vi "CAN Main.vi"(8 "error in (no error)":errorcluster, 10 "Interface":refnum<k21>="CAN1", 11 "Sequence Context In":refnum<k7>) -> (0 "error out":errorcluster)   [LabVIEW 2021, in "CAN wrapper.lvlib"]
uses:
  CAN wrapper.lvlib
  Private Controls/CAN States.ctl
  Private Controls/Setting.ctl
  <vilib>/addons/TestStand/_TSUtility.llb/TestStand - Set Property Value (Numeric Array).vi
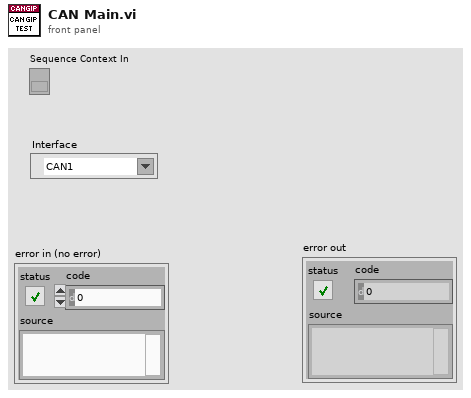
[diagram p1: front panel]
types:
  T1 = typedef "CAN wrapper.lvlib/CAN States.ctl" = enum16{"Init", "Rx Sess", "Tx Sess", "Read Signals", "Write Signals", "Close"}
  T2 = typedef "CAN wrapper.lvlib/Setting.ctl" = cluster{"Termination":u32, "Baud Rate":u64, "Interface":refnum<k21>, "XNET Database":refnum<k21>, "ECU":refnum<k21>}
  T3 = typedef "TestStand - Status Monitor.ctl" = cluster{"Sequence Context":refnum<k7>, "Execution":refnum<k7>, "Termination Monitor":refnum<k7>}
  T4 = cluster{"Send Tx":bool, "Stop":bool, "Rx Signals":string[], "Tx Signals":string[], "Tx Values In":dbl[]}
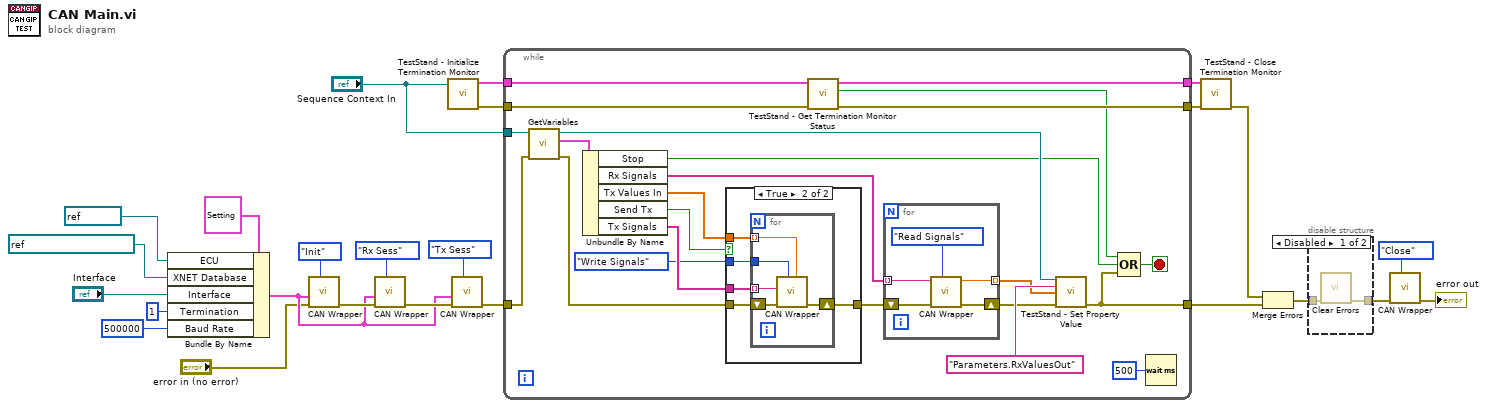
[diagram p0: block diagram]
diagram:
  n1 = Bundle By Name(cluster=T2 {"Termination"=1, "Baud Rate"=125000, "Interface"="CAN1", "XNET Database"="GIP_CAN_Database", "ECU"="GIP\nGIP_CAN_Database"} ("Setting"), "ECU"=refnum<k21> "GIP\ncan_messages_818", "XNET Database"=refnum<k21> "can_messages_818", "Interface"="Interface", "Termination"=u32 1, "Baud Rate"=u64 500000) -> (w13:T2)
  n2 = call "CAN Wrapper.vi"("States"=CAN_States."Init" ("CAN States"), "error in"="error in (no error)", "Setting"=w13) -> ("error out"=w24:errorcluster)  [unwired: 7 in, 1 out]
  n3 = call "CAN Wrapper.vi"("States"=CAN_States."Rx Sess" ("CAN States"), "error in"=w24, "Setting"=w13) -> ("error out"=w16:errorcluster)  [unwired: 7 in, 1 out]
  n4 = call <vilib>:"TestStand - Initialize Termination Monitor.vi"("Sequence Context In"="Sequence Context In") -> ("error out"=w10:errorcluster, "Status Monitor Out"=w9:T3)  [unwired: 9 in]
  n5 = call "CAN Wrapper.vi"("States"=CAN_States."Tx Sess", "error in"=w16, "Setting"=w13) -> ("error out"=w15:errorcluster)  [unwired: 7 in, 1 out]
  n6 = while {
    tunnel: w15 -> [w41]
    tunnel: w10 -> [w48]
    tunnel: w9 -> [w47]
    tunnel: [w46] -> w4
    tunnel: [w45] -> w7
    tunnel: "Sequence Context In" -> [w40]
    tunnel: [w34] -> w5
    stop <- w44 stop-if-true
    n7 = call "GetVariables.vi"("error in (no error)"=w41, "Sequence Context In"=w40) -> ("error out"=w38:errorcluster, "Variables"=w37:T4, "Sequence Context Out"=w39:refnum<k7>)  [unwired: 7 in]
    n8 = Unbundle By Name(w37) -> ("Stop"=w35:bool, "Rx Signals"=w27:string[], "Tx Values In"=w36:dbl[], "Send Tx"=w31:bool, "Tx Signals"=w32:string[])
    n9 = case shown="True" w31 {
      tunnel: w38 -> [w49 w54]
      tunnel: [w49 w51] -> w30
      tunnel: w32 -> [_ w52]
      tunnel: w36 -> [_ w53]
      tunnel: CAN_States."Write Signals" ("CAN States") -> [_ w50]
      frame False {
      }
      frame True {
        n10 = for {
          tunnel: w53 -> [w57] mode=indexing
          tunnel: w50 -> [w56]
          shift-right: [w58] -> w51
          shift-left: w54 -> [w59]
          tunnel: w52 -> [w55] mode=indexing
          n11 = call "CAN Wrapper.vi"("Signal Write"=w57, "States"=w56, "error in"=w59, "Tx Signal In"=w55) -> ("error out"=w58:errorcluster)  [unwired: 6 in, 1 out]
        }
      }
    }
    n12 = call <vilib>:"TestStand - Get Termination Monitor Status.vi"("error in (no error)"=w48, "Status Monitor In"=w47) -> ("error out"=w46:errorcluster, "Terminating or Aborting"=w43:bool, "Status Monitor Out"=w45:T3)  [unwired: 7 in]
    n13 = for {
      tunnel: w27 -> [w62] mode=indexing
      tunnel: [w61] -> w26 mode=indexing
      shift-right: [w63] -> w29
      shift-left: w30 -> [w64]
      n14 = call "CAN Wrapper.vi"("States"=CAN_States."Read Signals" ("CAN States"), "error in"=w64, "Rx Signal In"=w62) -> ("error out"=w63:errorcluster, "Signal out"=w61:dbl)  [unwired: 7 in]
    }
    n15 = call-poly <vilib>:"TestStand - Set Property Value.vi"("Sequence Context In"=w39, "Lookup String"="Parameters.RxValuesOut", "New Value"=w26, "error in (no error)"=w29) -> ("error out"=w34:errorcluster)  [unwired: 10 in, 1 out]
    n16 = Compound Arithmetic op=OR(w43, w35, w34) -> (w44:bool)
    n17 = Wait (ms)(milliseconds to wait=u32 500) -> ()  [unwired: 1 out]
  }
  n18 = call <vilib>:"TestStand - Close Termination Monitor.vi"("error in (no error)"=w4, "Status Monitor In"=w7) -> ("error out"=w3:errorcluster)  [unwired: 9 in]
  n19 = Merge Errors(w3, w5) -> (w8:errorcluster)
  n20 = disable-structure shown="Disabled" {
    disable-tunnel: w8 -> [w66 w67]
    disable-tunnel: [w65 w67] -> w1
    frame Disabled {
      n21 = call <vilib>:"Clear Errors.vi"("error in (no error)"=w66) -> ("error out"=w65:errorcluster)  [unwired: 5 in, 1 out]
    }
    frame Enabled {
    }
  }
  n22 = call "CAN Wrapper.vi"("States"=CAN_States."Close" ("CAN States"), "error in"=w1) -> ("error out"=→"error out":errorcluster)  [unwired: 8 in, 1 out]
